vi "putFactor.vi"(8 "error in":errorcluster, 10 "Exposure Factor":i32=1 caption="(01-15)", 11 "VISA in":refnum<visa-resource-name>="ASRL13::INSTR") -> (0 "error out":errorcluster, 1 "Status":bool, 3 "VISA out":refnum<visa-resource-name>="ASRL13::INSTR")   [LabVIEW 2025]
doc: "This VI is to select Sequence Mode.\n\nInput:\n- Sequence Mode:\n All : Set all channel to sequence mode.\n Single : Set only 1 channel to sequence mode.\n\nOutput:\n- Status:\n True : Passed\n False : Failed"
uses:
  <vilib>/Utility/error.llb/Trim Whitespace One-Sided.vi
panel:
  # "The exposure time will be increased when the factor isincreased which will lead to longer test times i.e. Factor 02 will double the test time, factor 03will treble the test time etc."
  # "Factory default setting: 01"
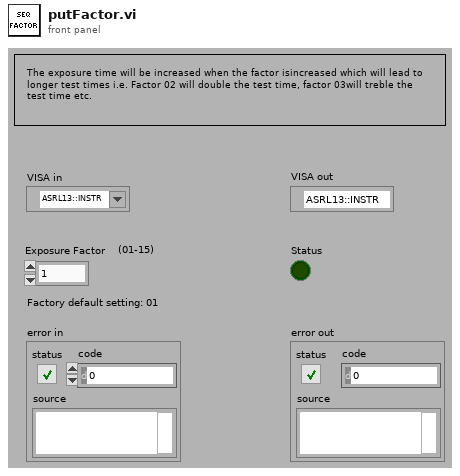
[diagram p1: front panel]
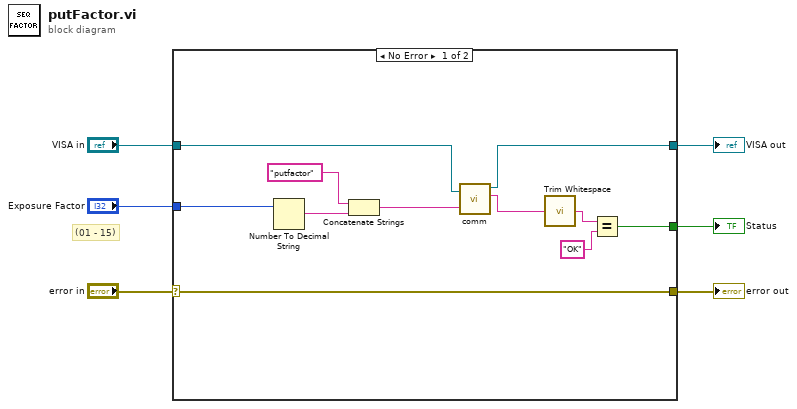
[diagram p0: block diagram]
diagram:
  # "(01 - 15)"
  n1 = case shown="No Error" "error in" {
    selector: "error in" -> [w8 w18]
    tunnel: "VISA in" -> [w17 _]
    tunnel: [w14 _] -> w5
    tunnel: "Exposure Factor" -> [w7 _]
    tunnel: [w9 _] -> w3
    tunnel: [w8 w18] -> w1
    frame No Error {
      n2 = Number To Decimal String(number=w7) -> (decimal integer string=w13:string)  [unwired: 1 in]
      n3 = Concatenate Strings("putfactor" ("Substring"), w13) -> (w16:string)
      n4 = call "comm.vi"("VISA resource name"=w17, "Command"=w16) -> ("dup VISA resource name"=w14:refnum<visa-resource-name>, "Response"=w12:string)  [unwired: 2 out]
      n5 = call <vilib>:"Trim Whitespace.vi"("string"=w12) -> ("trimmed string"=w11:string)  [unwired: 1 in]
      n6 = Equal?(x=w11, y="OK") -> (x = y?=w9:bool)
    }
    frame Error {
    }
  }
  "VISA out" <- w5
  "Status" <- w3
  "error out" <- w1
